vi "domeshmmonitorCommandCloseShutter.vi"(8 "error in (no error)":errorcluster, 11 "command_CloseShutter_Ctl":T1) -> (0 "error out":errorcluster, 2 "function return":i32, 3 "command_CloseShutter_Ctl out":T1)   [LabVIEW 2015, in "SALLV_dome.lvlib"]
doc: "int dome_shm_monitorCommand_CloseShutterLV(dome_command_CloseShutterLV *command_CloseShutter_Ctl );"
uses:
  SALLV_dome.lvlib
  SALLV_dome.so
  DataTypes/command_CloseShutter.ctl
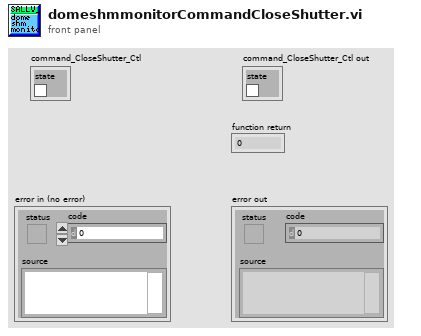
[diagram p1: front panel]
types:
  T1 = typedef "SALLV_dome.lvlib/command_CloseShutter.ctl" = cluster{"state":bool}
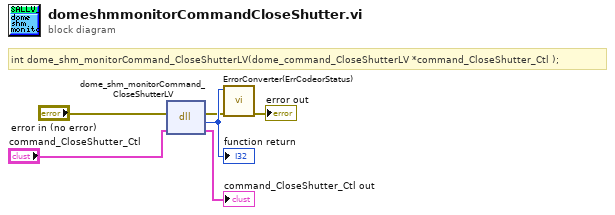
[diagram p0: block diagram]
diagram:
  # "int dome_shm_monitorCommand_CloseShutterLV(dome_command_CloseShutterLV *command_CloseShutter_Ctl );"
  n1 = dll-call lib="home/andres/Desktop/SALLV_dome2015/SALLV_dome.*" fn="dome_shm_monitorCommand_CloseShutterLV"(error in="error in (no error)", "command_CloseShutter_Ctl"="command_CloseShutter_Ctl") -> (error out=w2:errorcluster, w6:i32, "command_CloseShutter_Ctl"=→"command_CloseShutter_Ctl out":T1)  [unwired: 2 in, 1 out]
  "function return" <- w6
  n2 = call "ErrorConverter(ErrCodeorStatus).vi"("error in (no error)"=w2, "error code"=w6) -> ("error out"=→"error out":errorcluster)  [unwired: 9 in]
